vi "CMI ADS127L21 - Test.vi"() -> ()   [LabVIEW 2020]
uses:
  CMI ADS127L21 - Session.ctl
  CMI ADS127L21 - Input Range.ctl
  CMI ADS127L21 - Input Mode.ctl
  CMI ADS127L21 - Input Impedance.ctl
  CMI ADS127L21 - Record Channel.ctl
panel:
  out "FIFO usage [%]":dbl format="%.1f"
  out "record number":i32
  in  "Use External Source? (False: Internal)":bool
  in  "Channels":T1[](array[typedef])=[{"Range"=enum."±1.65V", "Channel"=1, "Mode"=enum."Normal", "Impedance"=enum."1M"}, {"Range"=enum."±1.65V", "Channel"=2, "Mode"=enum."Normal", "Impedance"=enum."1M"}] {"Channel" min=1 max=8 step=1}
  in  "stop records loop":bool
  in  "records count":i32=1
  out "FIFO transfer":i32
  out "timestamp [s]":dbl
  out "idn string":string
  in  "Sampling rate [Hz]":dbl=400000.0
  out "Waveform Graph":dbl[][](graph)
  out "error out":errorcluster
  out "sample data":dbl[][](array[numeric])
  in  "Samples Count (1000)":i32=1000
  in  "session in":T5 {"channels"."Channel" min=1 max=8 step=1}
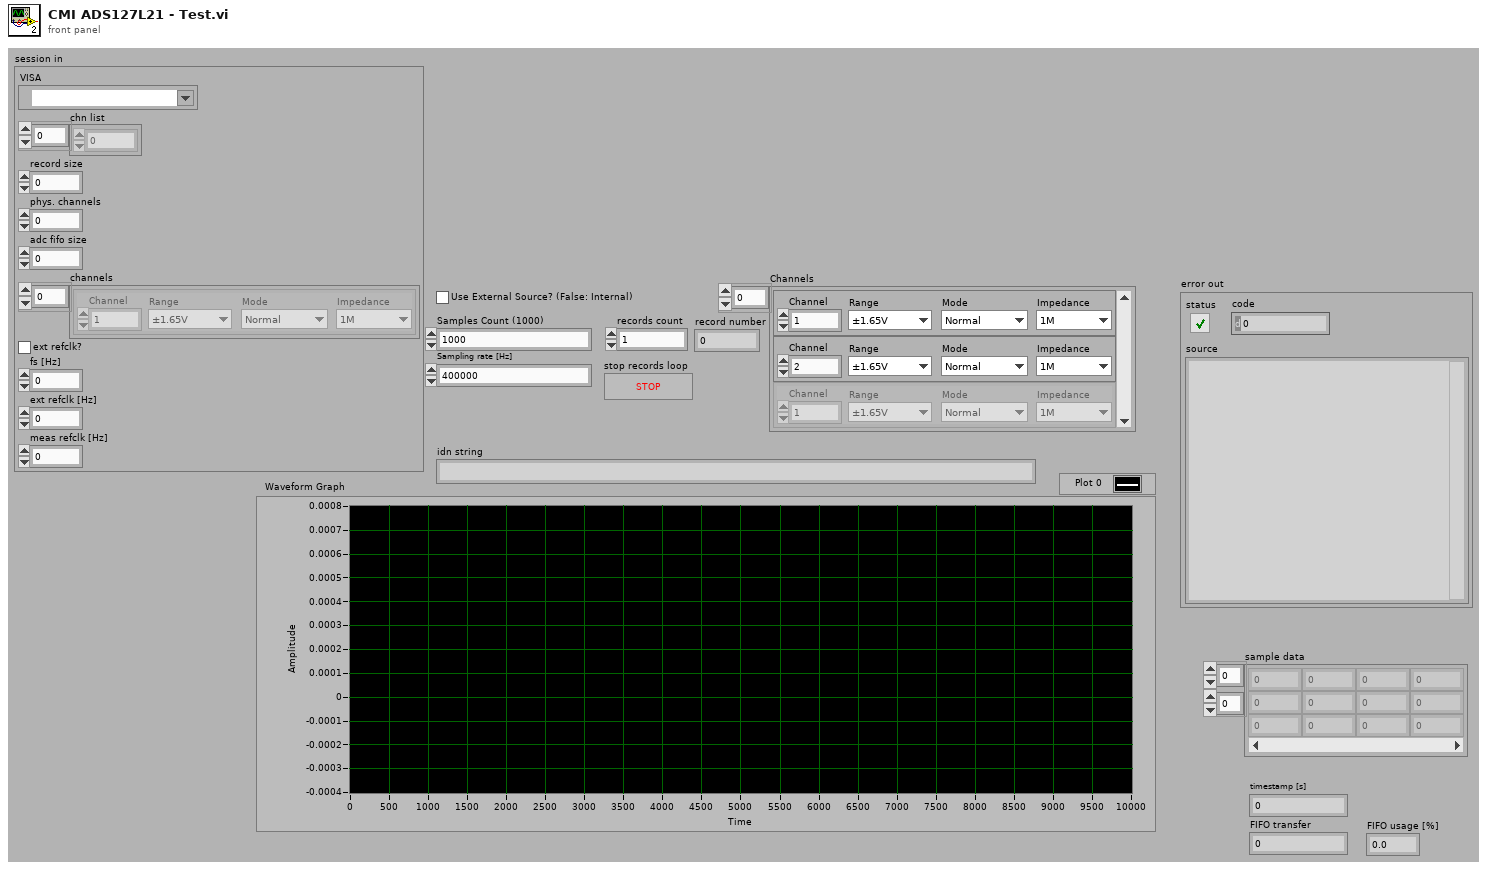
[diagram p1: front panel]
types:
  T1 = typedef "CMI ADS127L21 - Record Channel.ctl" = cluster{"Range":T2, "Channel":i32, "Mode":T3, "Impedance":T4}
  T2 = typedef "CMI ADS127L21 - Input Range.ctl" = enum16{"±1.65V", "±2V"}
  T3 = typedef "CMI ADS127L21 - Input Mode.ctl" = enum16{"Normal", "Inverted", "GND"}
  T4 = typedef "CMI ADS127L21 - Input Impedance.ctl" = enum16{"1M", "1k5"}
  T5 = typedef "CMI ADS127L21 - Session.ctl" = cluster{"VISA":refnum<visa-resource-name>, "chn list":i32[], "record size":i32, "phys. channels":i32, "adc fifo size":i32, "channels":T1[], "ext refclk?":bool, "fs [Hz]":dbl, "ext refclk [Hz]":dbl, "meas refclk [Hz]":dbl}
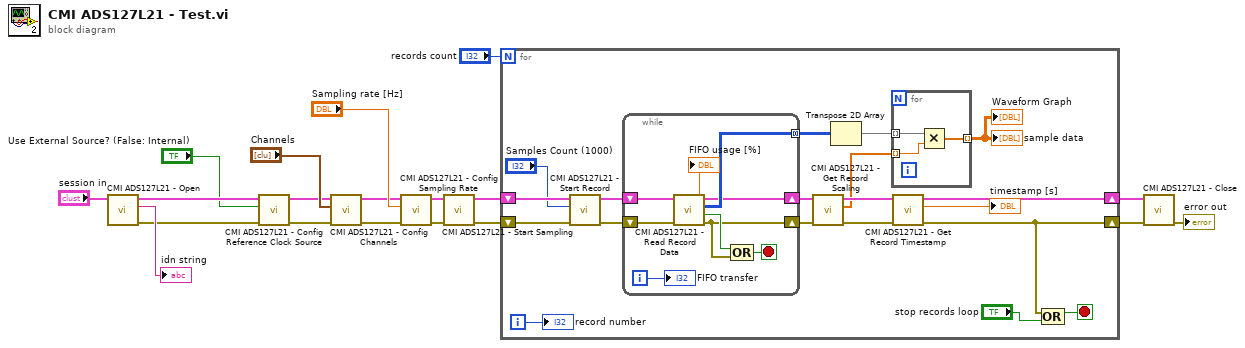
[diagram p0: block diagram]
diagram:
  n1 = call "CMI ADS127L21 - Open.vi"("session in"="session in") -> ("error out"=w5:errorcluster, "idn string"=→"idn string":string, "session out"=w2:T5)  [unwired: 8 in]
  n2 = call "CMI ADS127L21 - Config Reference Clock Source.vi"("error in (no error)"=w5, "Use External Source? (False: Internal)"="Use External Source? (False: Internal)", "session in"=w2) -> ("error out"=w4:errorcluster, "session out"=w3:T5)  [unwired: 7 in]
  n3 = call "CMI ADS127L21 - Config Channels.vi"("error in (no error)"=w4, "Channels"="Channels", "session in"=w3) -> ("error out"=w7:errorcluster, "session out"=w8:T5)  [unwired: 7 in]
  n4 = call "CMI ADS127L21 - Config Sampling Rate.vi"("error in (no error)"=w7, "Sampling rate [Hz]"="Sampling rate [Hz]", "session in"=w8) -> ("error out"=w12:errorcluster, "session out"=w13:T5)  [unwired: 7 in]
  n5 = call "CMI ADS127L21 - Start Sampling.vi"("error in (no error)"=w12, "session in"=w13) -> ("error out"=w18:errorcluster, "session out"=w17:T5)  [unwired: 8 in]
  n6 = for {
    N: "records count" -> [_]
    shift-right: [w20] -> w16
    shift-left: w18 -> [w38]
    shift-right: [w27] -> w15
    shift-left: w17 -> [w37]
    i -> [w23]
    stop <- w22 stop-if-true
    n7 = call "CMI ADS127L21 - Start Record.vi"("error in (no error)"=w38, 10:"Samples Count (1000)", "session in"=w37) -> ("error out"=w35:errorcluster, "session out"=w36:T5)  [unwired: 7 in]
    n8 = while {
      tunnel: [w46] -> w29 mode=concatenating
      shift-right: [w45] -> w33
      shift-left: w35 -> [w49]
      shift-right: [w44] -> w32
      shift-left: w36 -> [w50]
      i -> [w43]
      stop <- w47 stop-if-true
      n9 = call "CMI ADS127L21 - Read Record Data.vi"("error in (no error)"=w49, "session in"=w50) -> ("error out"=w45:errorcluster, "done?"=w48:bool, "Raw Sample Data (column per channel)"=w46:i32[][], "session out"=w44:T5, "FIFO usage [%]"=→"FIFO usage [%]":dbl)  [unwired: 5 in]
      n10 = Compound Arithmetic op=OR(w48, w45) -> (w47:bool)
      "FIFO transfer" <- w43
    }
    n11 = call "CMI ADS127L21 - Get Record Scaling.vi"("error in (no error)"=w33, "session in"=w32) -> ("error out"=w31:errorcluster, "Gain (one value per channel)"=w28:dbl[], "session out"=w30:T5)  [unwired: 7 in]
    n12 = Transpose 2D Array(2D array=w29) -> (transposed array=w26:i32[][])
    n13 = for {
      tunnel: w26 -> [w41] mode=indexing
      tunnel: w28 -> [w40] mode=indexing
      tunnel: [w39] -> w25 mode=indexing
      n14 = Multiply(x=w41, y=w40) -> (x*y=w39:dbl[])
    }
    "sample data" <- w25
    "Waveform Graph" <- w25
    n15 = call "CMI ADS127L21 - Get Record Timestamp.vi"("error in (no error)"=w31, "session in"=w30) -> ("error out"=w20:errorcluster, "timestamp [s]"=→"timestamp [s]":ext, "session out"=w27:T5)  [unwired: 7 in]
    n16 = Compound Arithmetic op=OR(w20, "stop records loop") -> (w22:bool)
    "record number" <- w23
  }
  n17 = call "CMI ADS127L21 - Close.vi"("error in (no error)"=w16, "session in"=w15) -> ("error out"=→"error out":errorcluster)  [unwired: 9 in]
